vi "get 2nd result.vi"(9 "test item":string, 11 "itemClusters":T1) -> (3 "result string":string)   [LabVIEW 2011]
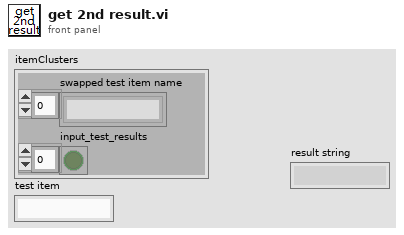
[diagram p1: front panel]
types:
  T1 = cluster{"swapped test item name":string[], "input_test_results":bool[]}
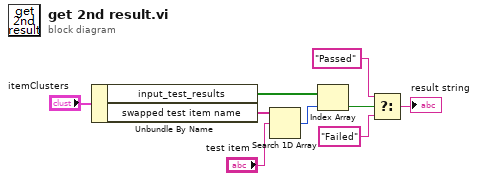
[diagram p0: block diagram]
diagram:
  n1 = Unbundle By Name("itemClusters") -> ("input_test_results"=w2:bool[], "swapped test item name"=w1:string[])
  n2 = Search 1D Array(1D array=w1, element="test item") -> (index of element=w8:i32)  [unwired: 1 in]
  n3 = Index Array(array=w2, index=w8) -> (element=w7:bool)
  n4 = Select(t="Passed", s=w7, f="Failed") -> (s? t:f=→"result string":string)
